vi "WPI_DualCameraSend Images To PC Loop.vi"(8 "error in (no error)":errorcluster, 10 "BackCameraDevRef":T1, 11 "FrontCameraDevRef":T1) -> ()   [LabVIEW 2016]
doc: "This VI is used to send images to the dashboard using the second enet port on the 8 slot controller. This is provided for compatibility, but is higher overhead than using the Camera MJPG approach.\n\nThis software is licensed. Open the labview\\readme\\WPI Robotics Library Open Source License.txt file for more information."
uses:
  <vilib>/Rock Robotics/SystemInterfaces/NetworkCommunication/NetComm_UsageReport_ResourceType.ctl
  <vilib>/vision/NI_Vision_Development_Module.lvlib
  Main/Robot Global Data.vi
  <vilib>/Rock Robotics/WPI/Camera/WPI_CameraDevRef.ctl
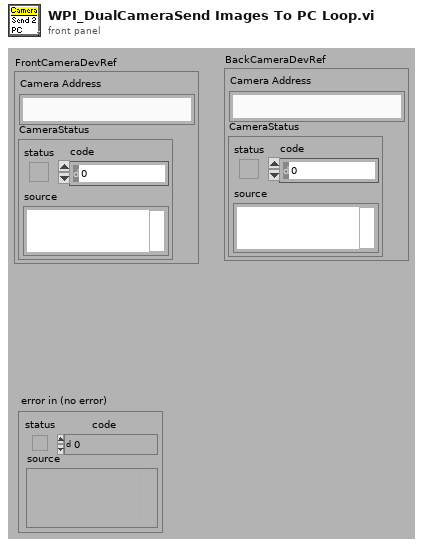
[diagram p1: front panel]
types:
  T1 = typedef "WPI_CameraDevRef.ctl" = cluster{"Camera Address":string, "CameraStatus":errorcluster}
  T2 = cluster{"fps":i32, "compression":i32, "compression 2":i32}
  T3 = typedef "NetComm_UsageReport_ResourceType.ctl" = enum8{"Controller", "Module", "Language", "CANPlugin", "Accelerometer", "ADXL345", "AnalogChannel", "AnalogTrigger", "AnalogTriggerOutput", "CANJaguar", "Compressor", "Counter", "Dashboard", "DigitalInput", "DigitalOutput", "DriverStationCIO", "DriverStationEIO", "DriverStationLCD", "Encoder", "GearTooth", "Gyro", "I2C", "Framework", "Jaguar", "Joystick", "Kinect", "KinectStick", "PIDController", "Preferences", "PWM", "Relay", "RobotDrive", "SerialPort", "Servo", "Solenoid", "SPI", "Task", "Ultrasonic", "Victor", "Button", "Command", "AxisCamera", "PCVideoServer", "SmartDashboard", "Talon", "HiTechnicColorSensor", "HiTechnicAccel", "HiTechnicCompass", "SRF08", "AnalogOutput", "Victor SP", "Talon SRX", "CAN Talon SRX", "ADXL362 Accel", "ADXRS450 Gyro", "Rev SPARK", "Mindsensors SD540", "Digital Filter", "ADIS16448", "PDP", "PCM", "PigeonIMU"}
  T4 = enum16{"Update Mode", "Get Image", "Get Image Data"}
  T5 = typedef "Image Type" = u32
  T6 = typedef "IMAQ Image.ctl" = refnum<image>
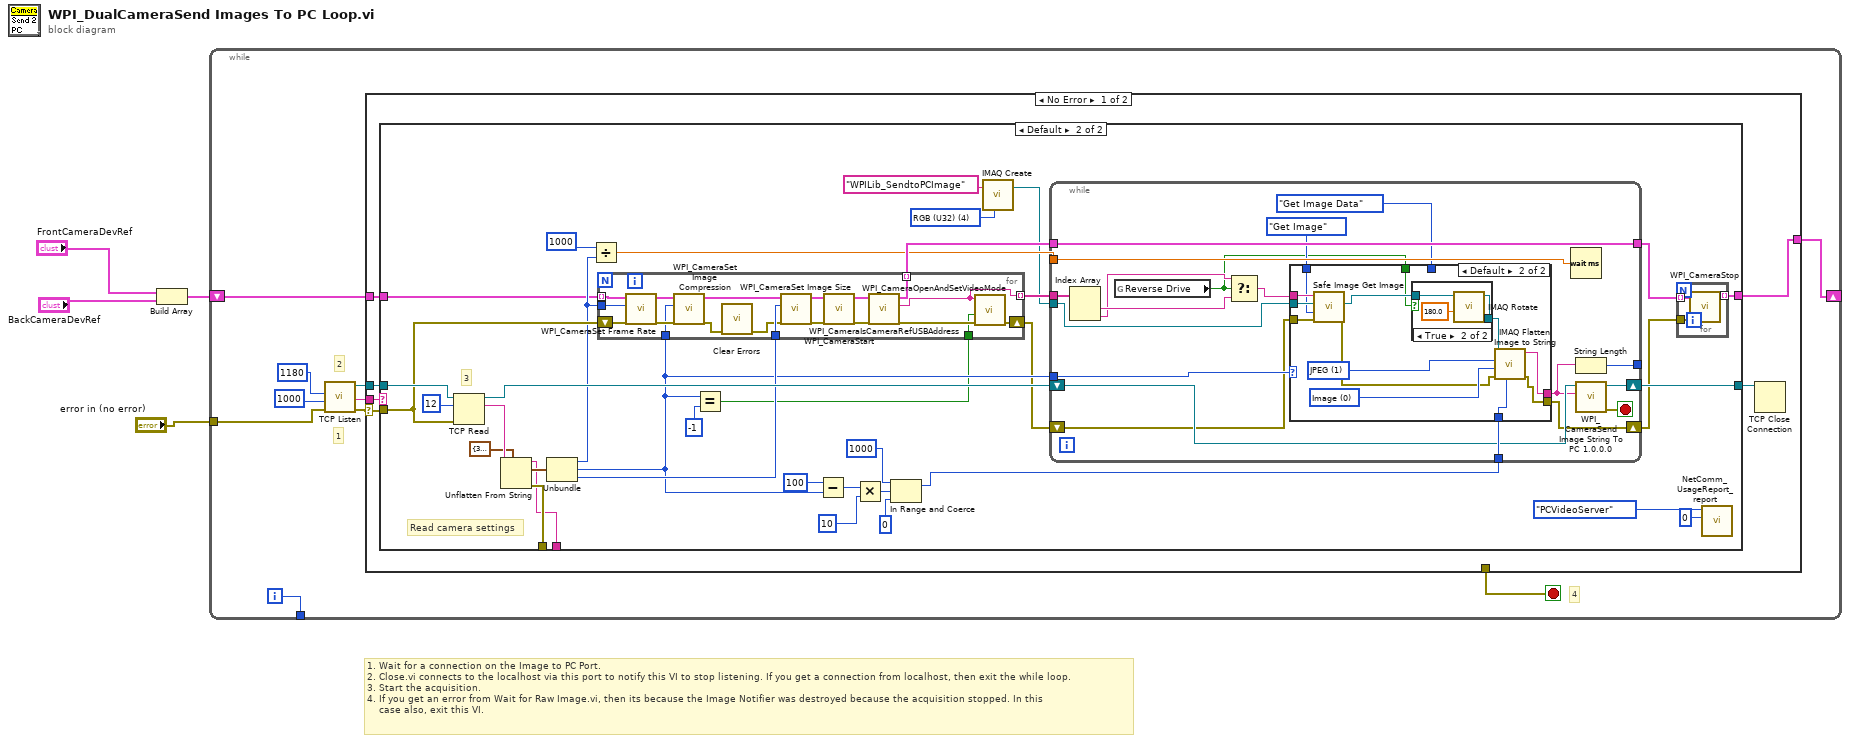
[diagram p0: block diagram]
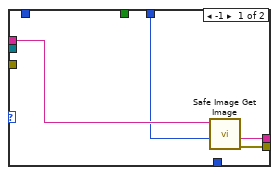
[diagram p3: hidden frame]
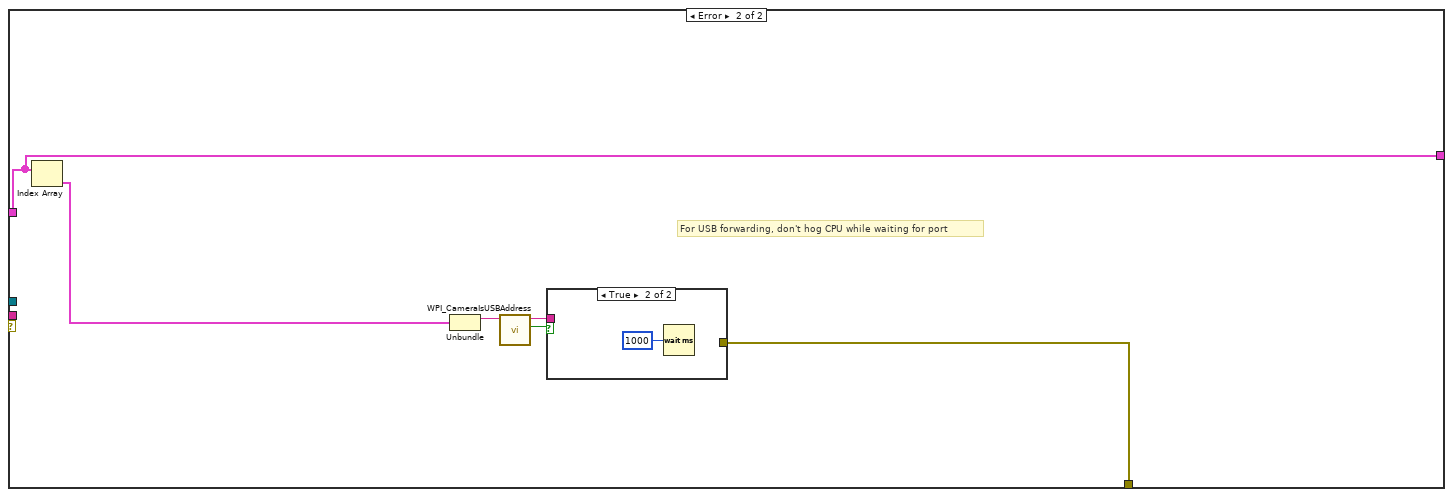
[diagram p5: hidden frame]
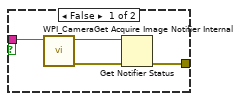
[diagram p6: hidden frame]
diagram:
  # "1. Wait for a connection on the Image to PC Port.\n2. Close.vi connects to the localhost via this port to notify this VI to stop listening. If you get a connection from localhost, then exit the while loop.\n3. Start the acquisition.\n4. If you get an error from Wait for Raw Image.vi, then its because the Image Notifier was destroyed because the acquisition stopped. In this\n    case also, exit this VI."
  n1 = Build Array("FrontCameraDevRef", "BackCameraDevRef") -> (w1:T1[])
  n2 = while {
    tunnel: "error in (no error)" -> [w13]
    tunnel: [w7] -> _
    shift-right: [w5] -> _
    shift-left: w1 -> [w6]
    i -> [w7]
    stop <- w11 stop-if-true
    # "4"
    # "1"
    # "2"
    n3 = call <vilib>:"TCP Listen.vi"("error in (no error)"=w13, "timeout ms (wait forever: -1)"=u16 1000 ("port"), "port"=u16 1180) -> ("error out"=w9:errorcluster, "remote address"=w14:string, "connection ID"=w12:refnum<k5>)  [unwired: 1 in, 5 out]
    n4 = case shown="No Error" w9 {
      selector: w9 -> [w17 _]
      tunnel: w14 -> [w20 _]
      tunnel: w12 -> [w19 _]
      tunnel: [_ w126] -> w11
      tunnel: w6 -> [w16 w121]
      tunnel: [w15 w121] -> w5
      frame No Error {
        n5 = case shown="Default" w20 {
          tunnel: w17 -> [_ w46]
          tunnel: w19 -> [w22 w50]
          tunnel: [w22 w58] -> w18
          tunnel: [_ w29] -> _
          tunnel: [_ w28] -> _
          tunnel: w16 -> [w21 w25]
          tunnel: [w21 w23] -> w15
          frame "localhost" {
          }
          frame Default {
            w53 = T5 4 items=["Grayscale (U8)", "Grayscale (I16)", "Grayscale (SGL)", "Complex (CSG)", "RGB (U32)", "HSL (U32)", "RGB (U64)", "Grayscale (U16)"] ("Image Type")
            # "Read camera settings"
            # "3"
            n6 = TCP Read(connection ID=w50, bytes to read=12, error in (no error)=w46) -> (connection ID out=w49:refnum<k5>, data out=w47:string)  [unwired: 2 in, 1 out]
            n7 = Unflatten From String(type=T2 {"fps"=30, "compression"=32, "compression 2"=32} ("Camera Settings"), binary string=w47) -> (rest of the binary string=w28:string, value=w45:T2, error out=w29:errorcluster)  [unwired: 3 in]
            n8 = Unbundle(w45) -> ("fps"=w42:i32, "compression"=w31:i32, "compression 2"=w44:i32)
            n9 = Divide(x=u16 1000 ("port"), y=w42) -> (x/y=w41:dbl)
            n10 = Equal?(x=w31, y=-1) -> (x = y?=w30:bool)
            n11 = for {
              tunnel: [w80] -> w52 mode=indexing
              tunnel: [w76] -> w51 mode=indexing
              tunnel: w44 -> [w69]
              tunnel: w42 -> [w68]
              tunnel: w31 -> [w67]
              tunnel: w30 -> [w66]
              shift-right: [w63] -> w26
              shift-left: w46 -> [w72]
              tunnel: w25 -> [w62] mode=indexing
              n12 = call <vilib>:"WPI_CameraSet Frame Rate.vi"("error in (no error)"=w72, "Frame Rate (fps)"=w68, "CameraDevRef"=w62) -> ("error out"=w71:errorcluster, "CameraDevRef Out"=w75:T1)  [unwired: 7 in]
              n13 = call <vilib>:"WPI_CameraSet Image Compression.vi"("error in (no error)"=w71, "Compression"=w67, "CameraDevRef"=w75) -> ("error out"=w65:errorcluster, "CameraDevRef Out"=w74:T1)  [unwired: 7 in]
              n14 = call <vilib>:"Clear Errors.vi"("error in (no error)"=w65) -> ("error out"=w64:errorcluster)  [unwired: 5 in, 1 out]
              n15 = call <vilib>:"WPI_CameraSet Image Size.vi"("error in (no error)"=w64, "Image Size"=w69, "CameraDevRef"=w74) -> ("error out"=w70:errorcluster, "CameraDevRef Out"=w73:T1)  [unwired: 7 in]
              n16 = call <vilib>:"WPI_CameraStart.vi"("error in (no error)"=w70, "CameraDevRef"=w73) -> ("error out"=w79:errorcluster, "CameraDevRef"=w77:T1)  [unwired: 8 out]
              n17 = call <vilib>:"WPI_CameraIsCameraRefUSBAddress.vi"("error in (no error)"=w79, "CameraDevRef"=w77) -> ("error out"=w78:errorcluster, "Camera Address Out"=w80:string, "CameraDevRef out"=w76:T1)  [unwired: 6 in, 1 out]
              n18 = call <vilib>:"WPI_CameraOpenAndSetVideoMode.vi"("error in (no error)"=w78, "USB JPEG"=w66, "Camera Address Out"=w80) -> ("error out"=w63:errorcluster)  [unwired: 8 in]
            }
            n19 = Subtract(x=100, y=w31) -> (x-y=w36:i32)
            n20 = Multiply(x=w36, y=10) -> (x*y=w38:i32)
            n21 = In Range and Coerce(upper limit=1000, x=w38, lower limit=0) -> (coerced(x)=w34:i32)  [unwired: 1 out]
            n22 = call "IMAQ Create"("Image Name"="WPILib_SendtoPCImage", "Image Type"=w53) -> ("New Image"=w27:T6)  [unwired: 3 in, 1 out]
            n23 = while {
              tunnel: w52 -> [w87]
              shift-right: [w99] -> w58
              shift-left: w49 -> [w93]
              tunnel: w27 -> [w98]
              tunnel: [w96] -> w57
              tunnel: w51 -> [w96]
              tunnel: w34 -> [w95]
              tunnel: w41 -> [w94]
              tunnel: [w91] -> _
              tunnel: w31 -> [w90]
              shift-right: [w82] -> w24
              shift-left: w26 -> [w83]
              stop <- w97 stop-if-true
              n24 = Index Array(array=w87) -> (element #1=w86:string, element #2=w85:string)  [unwired: 2 in]
              n25 = global read "Robot Global Data.vi" "Reverse Drive"() -> (w81:bool)
              n26 = Select(t=w85, s=w81, f=w86) -> (s? t:f=w84:string)
              n27 = case shown="Default" w90 {
                tunnel: [w102 w116] -> w92
                tunnel: w84 -> [w103 w112]
                tunnel: w98 -> [_ w111]
                tunnel: w95 -> [_ w113]
                tunnel: [w101 w105] -> w82
                tunnel: T4."Get Image Data" ("Operation") -> [w100 _]
                tunnel: T4."Get Image" ("Operation") -> [_ w110]
                tunnel: w83 -> [_ w107]
                tunnel: w81 -> [_ w104]
                frame -1 {
                  n28 = call <vilib>:"Safe Image Get Image.vi"("Operation"=w100, "Session In"=w103) -> ("error out"=w101:errorcluster, "Image Data String"=w102:string)  [unwired: 6 in, 2 out]
                }
                frame Default {
                  w114 = 0 items=["Image", "Image and Vision Info", "Reference to Image"] ("Type of Flatten (Image and Vision Info)")
                  w115 = 1 items=["None", "JPEG", "PACKED BINARY"] ("Compression (None)")
                  n29 = call <vilib>:"Safe Image Get Image.vi"("error in"=w107, "Operation"=w110, "Image In"=w111, "Session In"=w112) -> ("error out"=w106:errorcluster, "Image Out"=w109:T6)  [unwired: 4 in, 2 out]
                  n30 = case shown="True" w104 {
                    tunnel: w109 -> [w117 w120]
                    tunnel: [w117 w119] -> w108
                    frame False {
                    }
                    frame True {
                      n31 = call "IMAQ Rotate"("Angle (degrees)"=sgl 180.0, "Image Src"=w120) -> ("Image Dst Out"=w119:T6)  [unwired: 8 in, 1 out]
                    }
                  }
                  n32 = call "IMAQ Flatten Image to String"("Quality (750)"=w113, "error in (no error)"=w106, "Type of Flatten (Image and Vision Info)"=w114, "Compression (None)"=w115, "Image"=w108) -> ("error out"=w105:errorcluster, "Data String"=w116:string)  [unwired: 5 in]
                }
              }
              n33 = Wait (ms)(milliseconds to wait=w94) -> ()  [unwired: 1 out]
              n34 = String Length(string=w92) -> (length=w91:i32)
              n35 = call <vilib>:"WPI_CameraSend Image String To PC 1.0.0.0.vi"("String"=w92, "TCP Connection ID"=w93) -> ("error out"=w97:errorcluster, "TCP Connection ID out"=w99:refnum<k5>)  [unwired: 1 in, 7 out]
            }
            n36 = for {
              tunnel: w57 -> [w61] mode=indexing
              tunnel: w24 -> [w60]
              tunnel: [w59] -> w23 mode=indexing
              n37 = call <vilib>:"WPI_CameraStop.vi"("error in (no error)"=w60, "CameraDevRef"=w61) -> ("CameraDevRef"=w59:T1)  [unwired: 9 out]
            }
            n38 = call <vilib>:"NetComm_UsageReport_report.vi"("Instance Number"=u8 0, "Resource Type"=NetComm_UsageReport_ResourceType."PCVideoServer") -> ()  [unwired: 10 in]
          }
        }
        n39 = TCP Close Connection(connection ID=w18) -> ()  [unwired: 1 in, 3 out]
      }
      frame Error {
        # "For USB forwarding, don't hog CPU while waiting for port"
        n40 = Index Array(array=w121) -> (element=w123:T1)  [unwired: 1 in]
        n41 = Unbundle(w123) -> ("Camera Address"=w122:string)  [unwired: 1 out]
        n42 = call <vilib>:"WPI_CameraIsUSBAddress.vi"("Camera Address In"=w122) -> ("USB?"=w124:bool, "Camera Address Out"=w125:string)  [unwired: 8 in, 1 out]
        n43 = case shown="True" w124 {
          tunnel: [w130 _] -> w126
          tunnel: w125 -> [w127 _]
          frame False {
            n44 = call <vilib>:"WPI_CameraGet Acquire Image Notifier Internal.vi"("Camera Address"=w127) -> ("error out"=w128:errorcluster, "Acquire Image Notifier"=w129:refnum<notifier>)  [unwired: 1 in, 8 out]
            n45 = Get Notifier Status(notifier=w129, error in (no error)=w128) -> (error out=w130:errorcluster)  [unwired: 4 out]
          }
          frame True {
            n46 = Wait (ms)(milliseconds to wait=u32 1000) -> ()  [unwired: 1 out]
          }
        }
      }
    }
  }
